vi "LV terminals.vi"(8 "error in (no error)":errorcluster, 10 "Terms[]":refnum<vi>[](array[refnum]), 11 "String in":string) -> (0 "error out":errorcluster, 3 "String out":string)   [LabVIEW 2012]
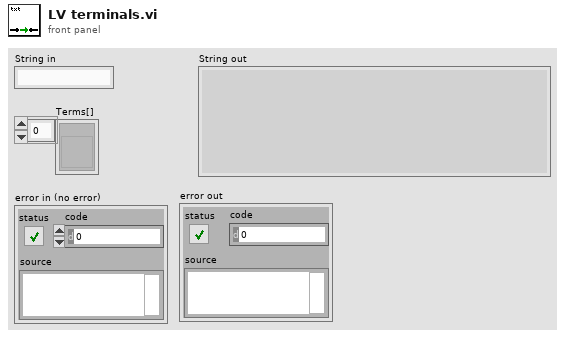
[diagram p1: front panel]
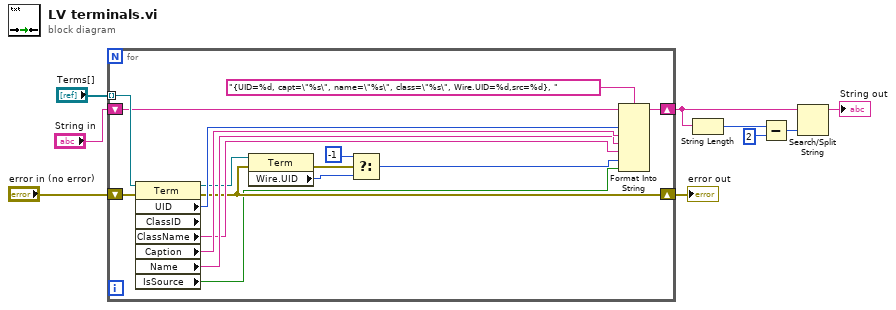
[diagram p0: block diagram]
diagram:
  n1 = for {
    tunnel: "Terms[]" -> [w25] mode=indexing
    shift-right: [w22] -> w3
    shift-left: "String in" -> [w23]
    shift-right: [w16] -> w1
    shift-left: "error in (no error)" -> [w18]
    n2 = property class="Term" props=["UID", "ClassID", "ClassName", "Caption", "Name", "IsSource"](reference=w25, error in=w18) -> (reference out=w17:refnum<vi>, error out=w16:errorcluster, "UID"=w24:i32, "ClassName"=w19:string, "Caption"=w21:string, "Name"=w20:string, "IsSource"=w15:bool)  [unwired: 1 out]
    n3 = property class="Term"(reference=w17, error in=w16) -> (error out=w13:errorcluster, "Wire.UID"=w11:i32)  [unwired: 1 out]
    n4 = Select(t=-1, s=w13, f=w11) -> (s? t:f=w10:i32)
    n5 = Format Into String(format string="{UID=%d, capt=\"%s\", name=\"%s\", class=\"%s\", Wire.UID=%d,src=%d}, ", initial string=w23, w24, w21, w20, w19, w10, w15) -> (resulting string=w22:string)  [unwired: 1 in, 1 out]
  }
  "error out" <- w1
  n6 = String Length(string=w3) -> (length=w4:i32)
  n7 = Subtract(x=w4, y=2) -> (x-y=w6:i32)
  n8 = Search/Split String(string=w3, offset (0)=w6) -> (substring before match=→"String out":string)  [unwired: 1 in, 2 out]
